vi "zadanie4.vi"() -> ()   [LabVIEW 2012]
panel:
  out "Obraz figur Lissajous":cluster{"Y":dbl[], "Y":dbl[]}[](graph)
  out "Użytkownik:":string
  in  "stop":bool
  in  "Wartość kąta a":dbl(knob) scale=0.0..90.0
  in  "Amplituda x = A":dbl
  in  "resetuj wejście x":bool
  in  "Wartość kąta b":dbl(knob) scale=0.0..90.0
  in  "Amplituda y = B":dbl
  in  "resetuj wejście y":bool
  in  "Naciśnij aby rozpocząć działanie programu":bool
  # "Program pozwala obserwować figury Lissajous.\nużytkownik może zmieniać wartość kątów, amplitudę i resetować wartości wejściowe."
  # "x(t) = A*sin(at)"
  # "y(t) = B*sin(bt)"
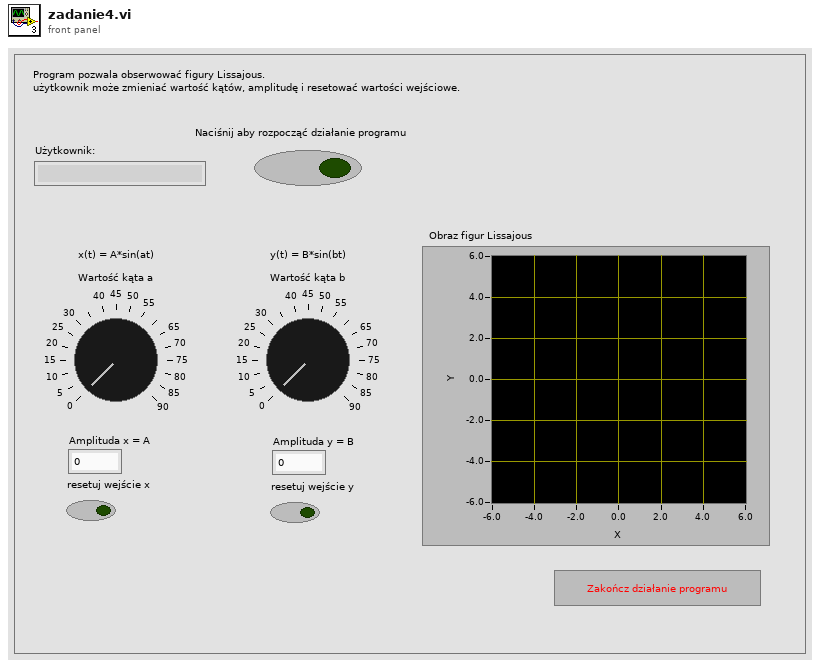
[diagram p1: front panel]
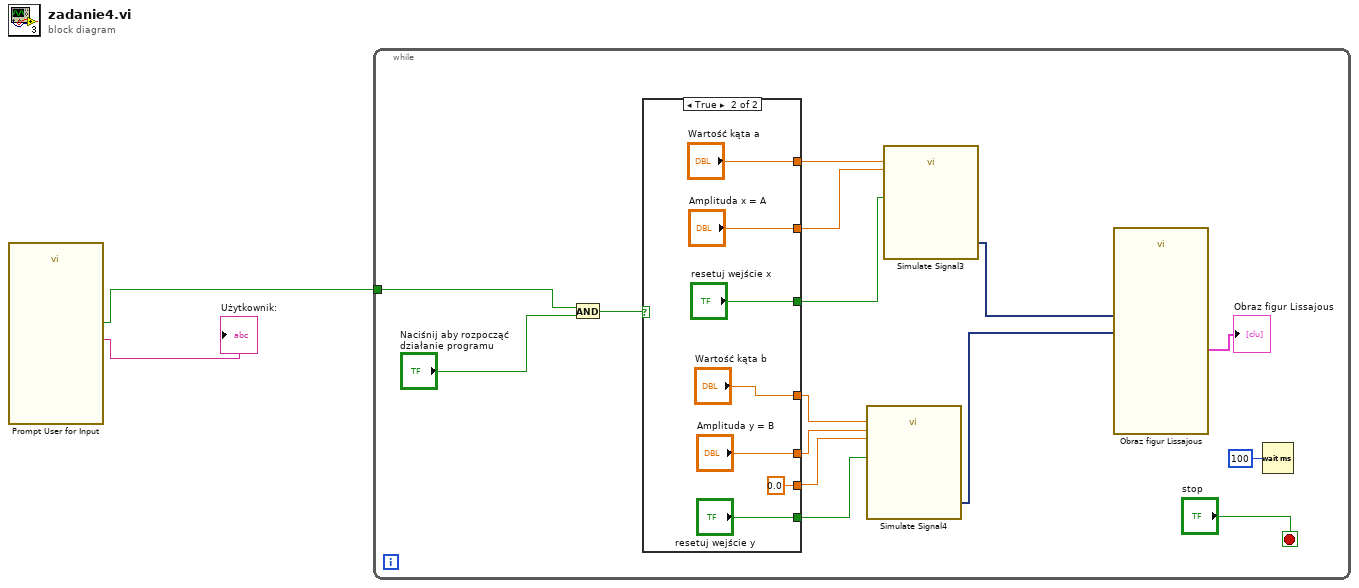
[diagram p0: block diagram]
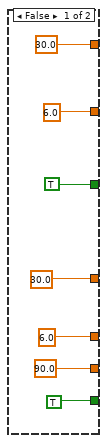
[diagram p2: hidden frame]
diagram:
  n1 = call "Prompt User for Input"() -> ("Nazwa użytkownika:"=→"Użytkownik:":string, "Dalej"=w1:bool)  [unwired: 16 in, 2 out]
  n2 = while {
    tunnel: w1 -> [w14]
    stop <- "stop" stop-if-true
    n3 = And(x=w14, y="Naciśnij aby rozpocząć działanie programu") -> (x .and. y?=w13:bool)
    n4 = case shown="True" w13 {
      tunnel: [TRUE ("reet_signal1") "resetuj wejście x"] -> w10
      tunnel: [6.0 ("Offset") "Amplituda x = A"] -> w11
      tunnel: [30.0 ("Frequency") "Wartość kąta a"] -> w12
      tunnel: [30.0 ("Offset") "Wartość kąta b"] -> w9
      tunnel: [6.0 ("Frequency") "Amplituda y = B"] -> w8
      tunnel: [TRUE ("reet_signal1") "resetuj wejście y"] -> w7
      tunnel: [90.0 ("Offset") 0.0 ("Offset")] -> w6
      frame False {
      }
      frame True {
      }
    }
    n5 = call "Simulate Signal4"("Reset Signal"=w7, "Frequency"=w9, "Amplitude"=w8, "Phase"=w6) -> ("Sinus b"=w3:dynamicdata)  [unwired: 10 in, 1 out]
    n6 = call "Simulate Signal3"("Reset Signal"=w10, "Frequency"=w12, "Amplitude"=w11) -> ("Sinus a"=w4:dynamicdata)  [unwired: 11 in, 1 out]
    n7 = call "Obraz figur Lissajous"("Y Input"=w3, "X Input"=w4) -> ("XY Graph"=→"Obraz figur Lissajous":cluster{"Y":dbl[], "Y":dbl[]}[])  [unwired: 3 in, 6 out]
    n8 = Wait (ms)(milliseconds to wait=u32 100) -> ()  [unwired: 1 out]
  }
